vi "FireBaseProyectoControlDePosicionPID.vi"() -> ()   [LabVIEW 2025]
uses:
  <vilib>/httpClient/PUTBuffer.vi
  <vilib>/httpClient/LabVIEWHTTPClient.lvlib
panel:
  in  "Tab Control":T1(tab)
  out "SetPoint":dbl
  out "Kp":dbl
  out "Ki":dbl
  out "Kd":dbl
  out "OutputPWM":dbl
  out "PosicionActual":dbl
  out "ContadorInterrupcion":dbl
  in  "SetPoint Ctrl":dbl
  in  "Kp Ctrl":dbl=0.8899999999999997 format="%03.3f"
  in  "Ki Ctrl":dbl=0.7560000000000003 format="%01.3f"
  in  "Kd Ctrl":dbl=0.43500000000000116 format="%01.3f"
  out "Body Desde el Servidor":string
  out "Header desde el servidor":string
  out "body hacia el servidor":string
  out "headers Hacia el Servidor":string
  out "Json Desde el Servidor":string
  out "Json al Servidor":string
  out "error out":errorcluster
  out "error out 2":errorcluster
  in  "stop":bool
  # "INTRUMENTACIoN VIRTUAL APLICADA"
  # "Control PID de un motor DC con conexión a FireBase"
  # "CONTROLES"
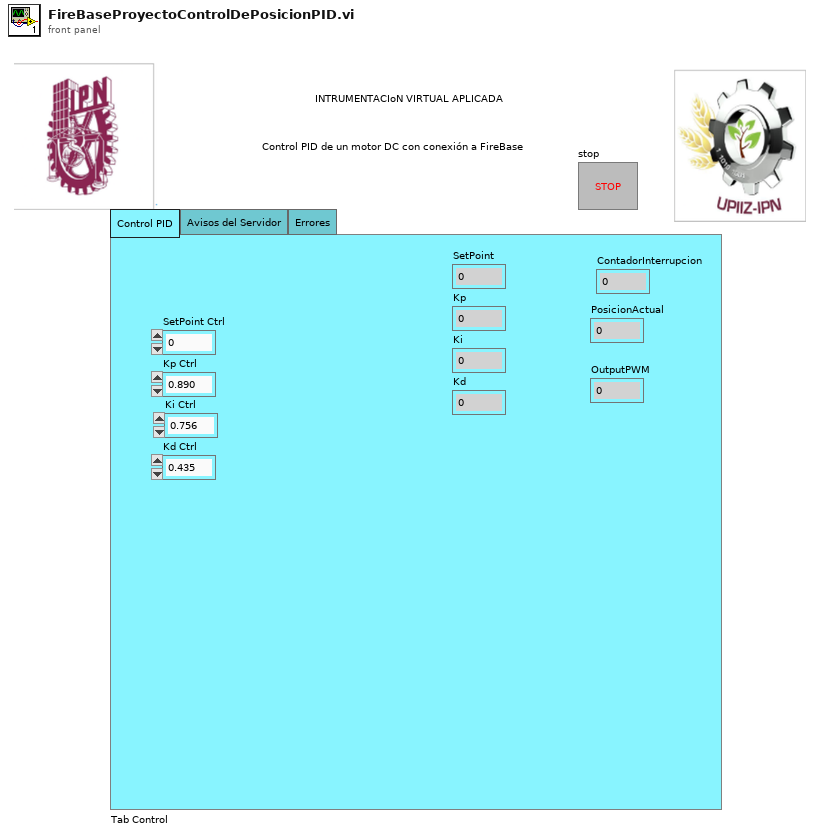
[diagram p1: front panel]
types:
  T1 = enum32{"Control PID", "Avisos del Servidor", "Errores"}
  T2 = cluster{"SetPoint":dbl, "Kp":dbl, "Ki":dbl, "Kd":dbl, "OutputPWM":dbl, "PosicionActual":dbl, "ContadorInterrupcion":dbl, "unstableVar":dbl}
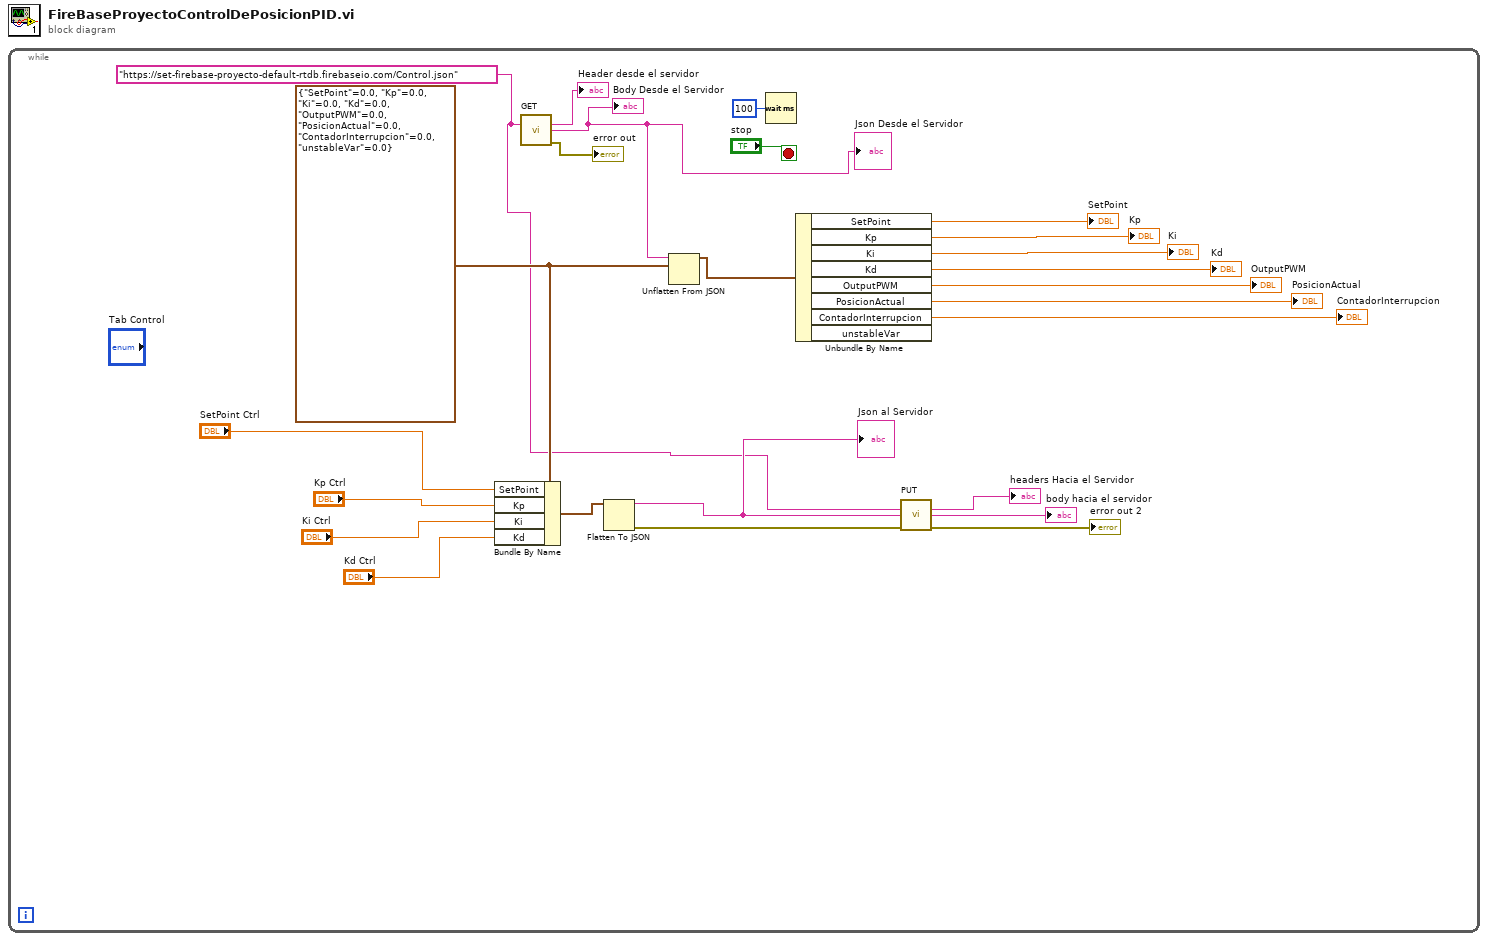
[diagram p0: block diagram]
diagram:
  n1 = while {
    stop <- "stop" stop-if-true
    w2 = T2 {"SetPoint"=0.0, "Kp"=0.0, "Ki"=0.0, "Kd"=0.0, "OutputPWM"=0.0, "PosicionActual"=0.0, "ContadorInterrupcion"=0.0, "unstableVar"=0.0}
    w1 = "https://set-firebase-proyecto-default-rtdb.firebaseio.com/Control.json" ("url")
    n2 = Bundle By Name "Bundle By Name"(cluster=w2, "SetPoint"="SetPoint Ctrl", "Kp"="Kp Ctrl", "Ki"="Ki Ctrl", "Kd"="Kd Ctrl") -> (w11:T2)
    n3 = call <vilib>:"GET.vi"("url"=w1) -> ("headers"=→"Header desde el servidor":string, "body"=w6:string, "error out"=→"error out":errorcluster)  [unwired: 11 in, 1 out]
    "Body Desde el Servidor" <- w6
    "Json Desde el Servidor" <- w6
    n4 = Flatten To JSON(anything=w11) -> (JSON string=w7:string, 11:w12:errorcluster)  [unwired: 2 in]
    "Json al Servidor" <- w7
    n5 = Unflatten From JSON(JSON string=w6, type and defaults=w2) -> (value=w21:T2)  [unwired: 5 in, 1 out]
    n6 = Wait (ms)(milliseconds to wait=u32 100) -> ()  [unwired: 1 out]
    n7 = Unbundle By Name "Unbundle By Name"(w21) -> ("SetPoint"=→"SetPoint":dbl, "Kp"=→"Kp":dbl, "Ki"=→"Ki":dbl, "Kd"=→"Kd":dbl, "OutputPWM"=→"OutputPWM":dbl, "PosicionActual"=→"PosicionActual":dbl, "ContadorInterrupcion"=→"ContadorInterrupcion":dbl)  [unwired: 1 out]
    n8 = call-poly <vilib>:"PUT.vi"("url"=w1, "buffer"=w7, "error in (no error)"=w12) -> ("headers"=→"headers Hacia el Servidor":string, "body"=→"body hacia el servidor":string, "error out"=→"error out 2":errorcluster)  [unwired: 9 in, 1 out]
  }
